vi "Clear Errors.vi"(4 "error in (no error)":errorcluster caption="Fehler (Eingang, kein Fehler)") -> (0 "error out":errorcluster caption="Fehler (Ausgang)")   [LabVIEW 2009]
doc: "In einem solchen Fall wird der Fehler-<B>Status</B> zu keinem Fehler, <B>Code</B> zu 0 und <B> Quelle</B> zu einem leeren String. Verwenden Sie dieses VI, wenn ein Fehler ignoriert werden soll."
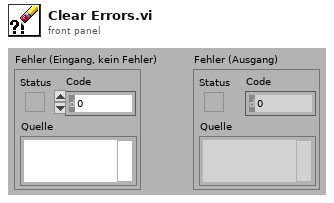
[diagram p1: front panel]
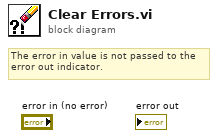
[diagram p0: block diagram]
diagram:
  # "The error in value is not passed to the\nerror out indicator."
